vi "Counter_SetFrequency.vi"(3 "error in (no error)":errorcluster, 4 "frequency":dbl, 5 "Task ID":u32) -> (0 "error out":errorcluster, 2 "Task ID":u32)   [LabVIEW 2015]
uses:
  Windows/System32/AdvLvDaq.dll
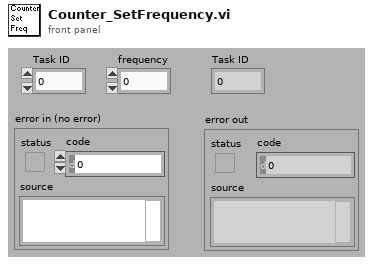
[diagram p1: front panel]
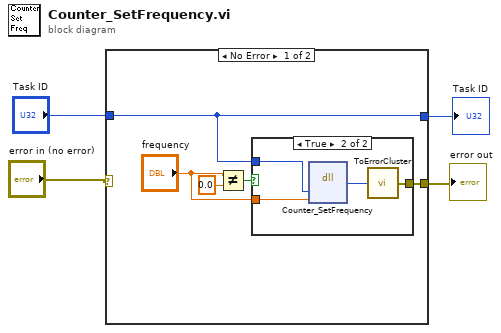
[diagram p0: block diagram]
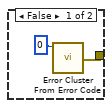
[diagram p2: hidden frame]
diagram:
  n1 = case shown="No Error" "error in (no error)" {
    selector: "error in (no error)" -> [_ w16]
    tunnel: "Task ID" -> [w7 w17]
    tunnel: [w7 w17] -> w2
    tunnel: [w5 w16] -> w1
    frame No Error {
      n2 = Not Equal?(x="frequency", y=0.0) -> (x != y?=w8:bool)
      n3 = case shown="True" w8 {
        tunnel: w7 -> [_ w15]
        tunnel: "frequency" -> [_ w14]
        tunnel: [w10 w12] -> w5
        frame False {
          n4 = call <vilib>:"Error Cluster From Error Code.vi"("error code (0)"=0) -> ("error out"=w10:errorcluster)  [unwired: 2 in, 6 out]
        }
        frame True {
          n5 = dll-call lib="C:/Windows/System32/AdvLvDaq.dll" fn="Counter_SetFrequency"("taskId"=w15, "frequency"=w14) -> ("return type"=w13:i32)  [unwired: 5 in, 2 out]
          n6 = call "ToErrorCluster.vi"("error code"=w13) -> ("error out"=w12:errorcluster)
        }
      }
    }
    frame Error {
    }
  }
  "Task ID" <- w2
  "error out" <- w1
